vi "Encoder Reset.vi"(8 "error in (no error)":errorcluster, 11 "DriveMotors in":refnum<class "DriveMotors.lvclass">) -> (0 "error out":errorcluster, 3 "DriveMotors out":refnum<class "DriveMotors.lvclass">)   [LabVIEW 2013, in "DriveMotors.lvclass"]
uses:
  DriveMotors.lvclass
  DriveMotors.lvclass/DriveMotors.ctl
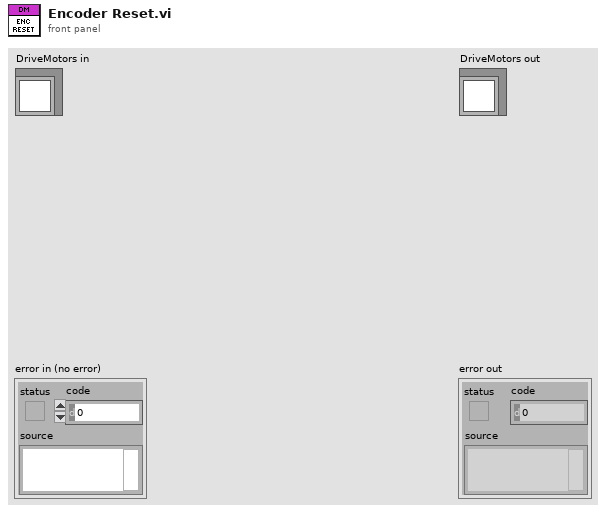
[diagram p1: front panel]
types:
  T1 = typedef "WPI_EncoderDevRef.ctl" = cluster{"DevStatus":errorcluster, "EncoderIndex":T2, "CounterIndex":T3, "DistancePerCount":dbl, "Decoding Type":T4}
  T2 = typedef "FPGA_EncoderIdx.ctl" = enum8{"Enc 0", "Enc 1", "Enc 2", "Enc 3", "Invalid"}
  T3 = typedef "FPGA_CounterCtrSystemIndex.ctl" = enum8{"Ctr 0", "Ctr 1", "Ctr 2", "Ctr 3", "Ctr 4", "Ctr 5", "Ctr 6", "Ctr 7", "Invalid"}
  T4 = typedef "WPI_EncoderType.ctl" = enum16{"1x", "2x", "4x"}
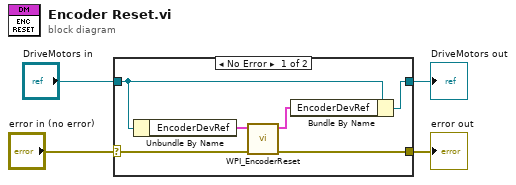
[diagram p0: block diagram]
diagram:
  n1 = case shown="No Error" "error in (no error)" {
    selector: "error in (no error)" -> [w8 w12]
    tunnel: [w7 w12] -> w3
    tunnel: [w6 w11] -> w1
    tunnel: "DriveMotors in" -> [w10 w11]
    frame No Error {
      n2 = Unbundle By Name(w10) -> ("EncoderDevRef"=w9:T1)
      n3 = call <vilib>:"WPI_EncoderReset.vi"("error in (no error)"=w8, "EncoderDevRef"=w9) -> ("error out"=w7:errorcluster, "EncoderDevRef"=w5:T1)  [unwired: 8 out]
      n4 = Bundle By Name(cluster=w10, "EncoderDevRef"=w5) -> (w6:refnum<class "DriveMotors.lvclass">)
    }
    frame Error {
    }
  }
  "error out" <- w3
  "DriveMotors out" <- w1
